vi "参考-my_onnx_test.vi"() -> ()   [LabVIEW 2022 SP3]
panel:
  out "运行时间":u32
  out "error out load":errorcluster
  out "error out object":errorcluster
  in  "OK Button":bool
  in  "关闭界面":bool
  in  "图片名":string
  out "模型名":string="deeplabv3_resnet101.onnx"
  out "error out":errorcluster
  out "程序路径名":path
  out "return value":i32
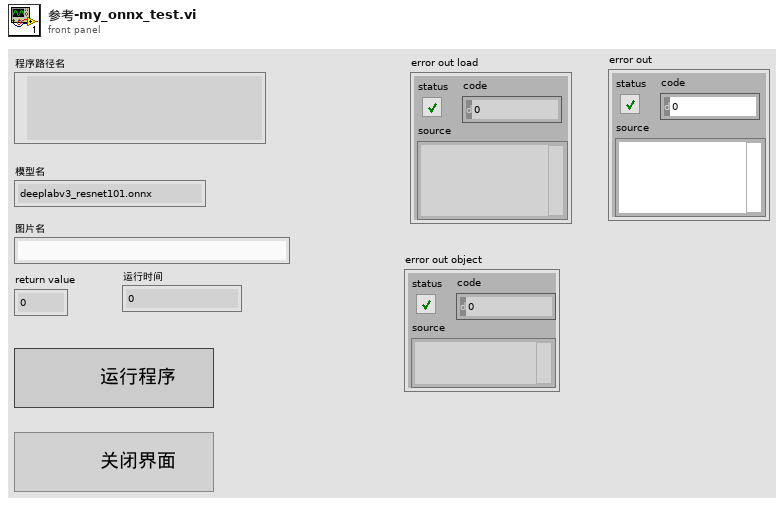
[diagram p1: front panel]
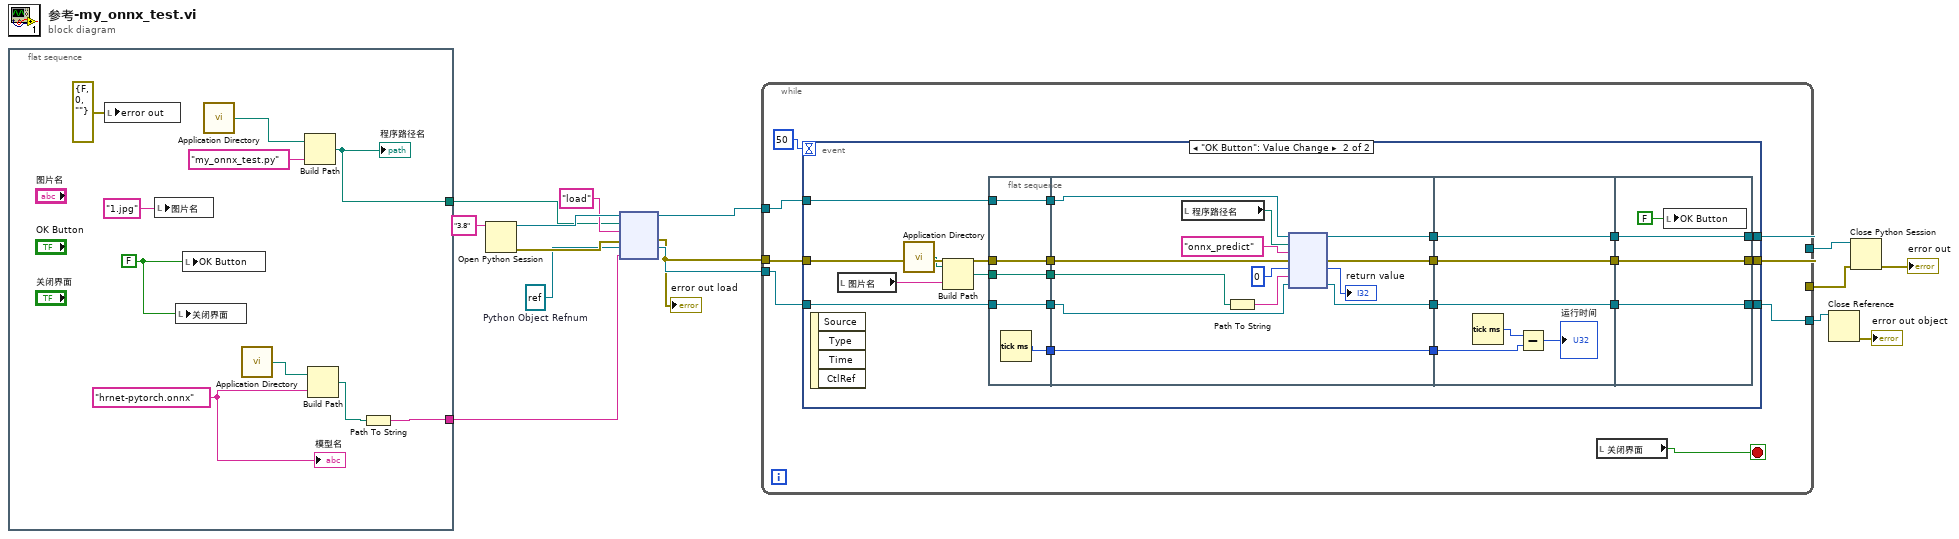
[diagram p0: block diagram]
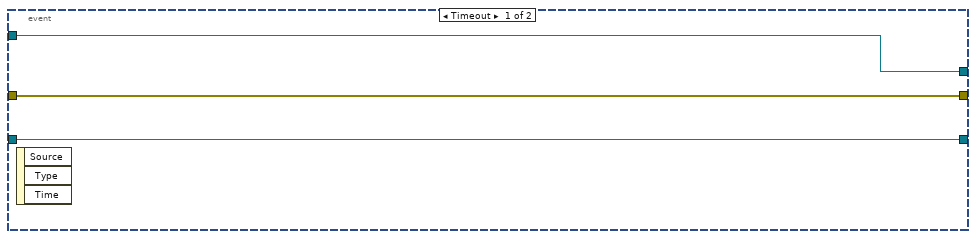
[diagram p2: hidden frame]
diagram:
  w8 = refnum<k38> refnum  # Python Object Refnum
  n1 = flat-sequence {
    tunnel: [w19] -> w2
    tunnel: [w16] -> w1
    frame #0 {
      w20 = "hrnet-pytorch.onnx"
      w24 = FALSE ("OK Button")
      n2 = local write "error out"(errorcluster {"status"=FALSE, "code"=0, "source"=""} ("error out")) -> ()
      n3 = local write "图片名"("1.jpg") -> ()
      n4 = local write "关闭界面"(w24) -> ()
      n5 = local write "OK Button"(w24) -> ()
      n6 = call <vilib>:"Application Directory.vi"() -> ("Application Directory"=w18:path)
      n7 = call <vilib>:"Application Directory.vi"() -> ("Application Directory"=w21:path)
      n8 = Build Path(base path=w18, name or relative path="my_onnx_test.py") -> (appended path=w16:path)
      "程序路径名" <- w16
      n9 = Build Path(base path=w21, name or relative path=w20) -> (appended path=w22:path)
      n10 = Path To String(path=w22) -> (string=w19:string)
      "模型名" <- w20
    }
  }
  n11 = Open Python Session(python version="3.8" ("Python version")) -> (session out=w11:refnum<k35>, error out=w9:errorcluster)  [unwired: 2 in]
  n12 = node(w11, w1, "load" ("function name"), w9, w8, w2) -> (w5:refnum<k35>, w6:errorcluster, w7:refnum<k38>)  [unwired: 1 in, 2 out]
  "error out load" <- w6
  n13 = while {
    tunnel: w5 -> [w31]
    tunnel: [w30] -> w13
    tunnel: [w29] -> w12
    tunnel: w6 -> [w28]
    tunnel: w7 -> [w27]
    tunnel: [w26] -> w4
    stop <- w33 stop-if-true
    n14 = event shown="[1] \"OK Button\": Value Change" {
      selector: _ -> [_ _]
      dyn-events: _ -> [_ _]
      timeout: 50 -> [_ _]
      tunnel: w31 -> [w36 w57]
      tunnel: [w36 w56] -> w30
      tunnel: [w35 w54] -> w29
      tunnel: w28 -> [w35 w52]
      tunnel: w27 -> [w34 w51]
      tunnel: [w34 w50] -> w26
      event Timeout {
        n15 = event-data() -> ()  [unwired: 1 in, 3 out]
      }
      event "OK Button": Value Change {
        n16 = event-data() -> ()  [unwired: 1 in, 4 out]
        n17 = local read "图片名"() -> (w46:string)
        n18 = call <vilib>:"Application Directory.vi"() -> ("Application Directory"=w47:path)
        n19 = Build Path(base path=w47, name or relative path=w46) -> (appended path=w45:path)
        n20 = flat-sequence {
          tunnel: w45 -> [w59]
          tunnel: w51 -> [w60]
          tunnel: w52 -> [w61]
          tunnel: w57 -> [w62]
          tunnel: [w62] -> w44
          tunnel: [w61] -> w43
          tunnel: [w60] -> w42
          tunnel: [w58] -> w41
          tunnel: [w59] -> w40
          tunnel: [w71] -> w55
          tunnel: [w70] -> w53
          tunnel: [w65] -> w49
          tunnel: [w64] -> w48
          tunnel: w44 -> [w72]
          tunnel: w43 -> [w69]
          tunnel: w42 -> [w67]
          tunnel: w41 -> [w64]
          tunnel: w40 -> [w63]
          tunnel: w55 -> [w81]
          tunnel: w53 -> [w80]
          tunnel: w49 -> [w79]
          tunnel: w48 -> [w77]
          tunnel: [w81] -> w39
          tunnel: [w80] -> w38
          tunnel: [w79] -> w37
          tunnel: [w83] -> w50
          tunnel: [w84] -> w54
          tunnel: [w85] -> w56
          tunnel: w39 -> [w85]
          tunnel: w38 -> [w84]
          tunnel: w37 -> [w83]
          frame #0 {
            n21 = Tick Count (ms)() -> (millisecond timer value=w58:u32)
          }
          frame #1 {
            n22 = local read "程序路径名"() -> (w68:path)
            n23 = Path To String(path=w63) -> (string=w75:string)
            n24 = node(w72, w68, "onnx_predict" ("function name"), w69, 0, w75, w67) -> (w71:refnum<k35>, w70:errorcluster, →"return value":i32, w65:refnum<k38>)  [unwired: 1 in, 2 out]
          }
          frame #2 {
            n25 = Tick Count (ms)() -> (millisecond timer value=w78:u32)
            n26 = Subtract(x=w78, y=w77) -> (x-y=→"运行时间":u32)
          }
          frame #3 {
            n27 = local write "OK Button"(FALSE ("OK Button")) -> ()
          }
        }
      }
    }
    n28 = local read "关闭界面"() -> (w33:bool)
  }
  n29 = Close Reference(reference=w4) -> (error out=→"error out object":errorcluster)  [unwired: 1 in]
  n30 = Close Python Session(session in=w13, error in=w12) -> (11:→"error out":errorcluster)
